vi "CreateXmlFromReadings.vi"() -> (1 "poziom":dbl(graph), 2 "natlenienie":dbl(graph), 3 "xml string":string)   [LabVIEW 2020]
uses:
  ProcessData.ctl
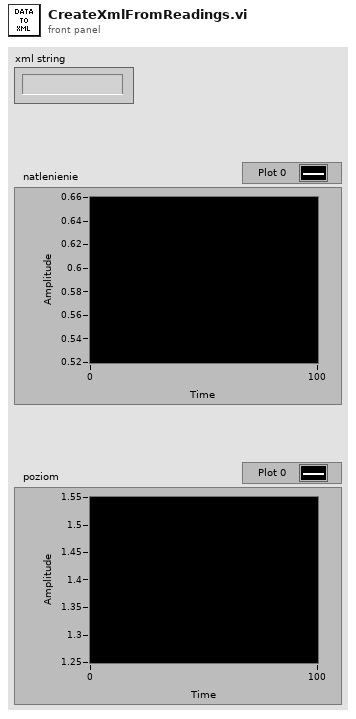
[diagram p1: front panel]
types:
  T1 = typedef "ProcessData.ctl" = cluster{"poziom":dbl, "natlenienie":dbl}
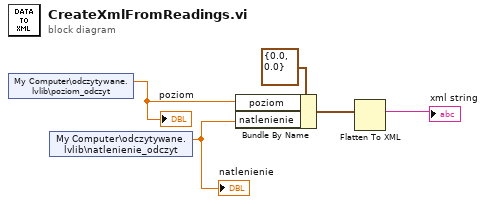
[diagram p0: block diagram]
diagram:
  n1 = shared-variable "My Computer\\odczytywane.lvlib\\poziom_odczyt"() -> (w3:dbl)  [unwired: 1 in, 1 out]
  "poziom" <- w3
  n2 = shared-variable "My Computer\\odczytywane.lvlib\\natlenienie_odczyt"() -> (w4:dbl)  [unwired: 1 in, 1 out]
  "natlenienie" <- w4
  n3 = Bundle By Name(cluster=T1 {"poziom"=0.0, "natlenienie"=0.0} ("Cluster"), "poziom"=w3, "natlenienie"=w4) -> (w1:T1)
  n4 = Flatten To XML(6:w1) -> (2:→"xml string":string)
